vi "ULx Create Channel (AI-Current-Basic).vi"(0 "task in":refnum<k24>, 1 "maximum value":dbl=2.5 format="%_4g", 2 "minimum value":dbl=0.5 format="%_4f", 5 "physical channels":refnum<k21>, 11 "error in":errorcluster) -> (4 "task out":refnum<k24>, 15 "error out":errorcluster)   [LabVIEW 2020]
doc: "Creates channel(s) to measure current."
uses:
  C:/Users/William/Documents/LV 2020 builds/LeaktestDAQ/Source-v33/ULx_LV.dll
  ULx_LV.dll
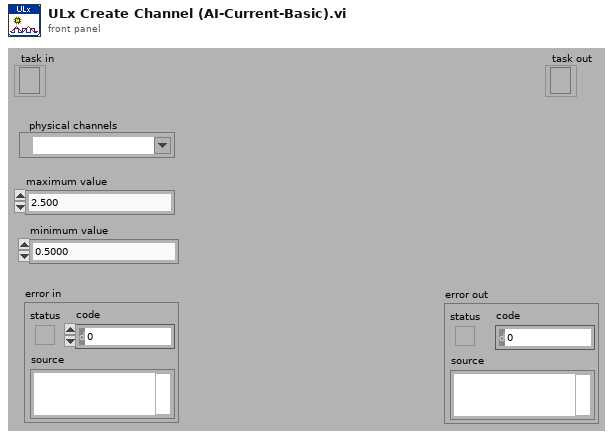
[diagram p1: front panel]
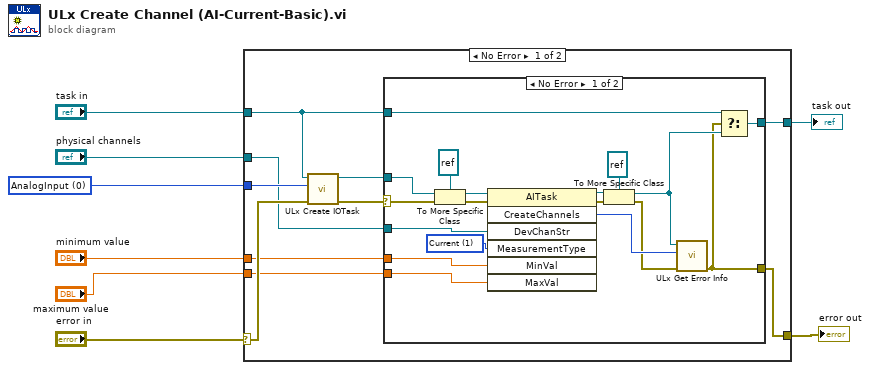
[diagram p0: block diagram]
diagram:
  w2 = 0 items=["AnalogInput", "AnalogOutput", "DigitalInput", "DigitalOutput", "CounterInput", "CounterOutput", "CompositeInput", "CompositeOutput", "TemperatureInput"] ("taskType")
  n1 = case shown="No Error" "error in" {
    selector: "error in" -> [w18 w40]
    tunnel: "task in" -> [w9 w39]
    tunnel: "physical channels" -> [w10 _]
    tunnel: w2 -> [w11 _]
    tunnel: [w16 w39] -> w6
    tunnel: [w15 w40] -> w5
    tunnel: "minimum value" -> [w13 _]
    tunnel: "maximum value" -> [w12 _]
    frame No Error {
      n2 = call "ULx Create IOTask.vi"("error in"=w18, "taskType"=w11, "i/o task in"=w9) -> ("error out"=w17:errorcluster, "i/o task out"=w14:refnum<k24>)  [unwired: 7 in]
      n3 = case shown="No Error" w17 {
        selector: w17 -> [w34 w38]
        tunnel: [w20 w38] -> w15
        tunnel: [w19 w37] -> w16
        tunnel: w14 -> [w32 _]
        tunnel: w10 -> [w31 _]
        tunnel: w13 -> [w29 _]
        tunnel: w12 -> [w28 _]
        tunnel: w9 -> [w22 w37]
        frame No Error {
          w27 = 1 items=["Voltage", "Current"] ("MeasurementType")
          n4 = To More Specific Class(target class=refnum<k24> refnum, reference=w32, error in=w34) -> (specific class reference=w35:refnum<k24>, error out=w33:errorcluster)
          n5 = invoke class="AITask" method="CreateChannels"(reference=w35, error in=w33, "DevChanStr"=w31, "MeasurementType"=w27, "MinVal"=w29, "MaxVal"=w28) -> (reference out=w25:refnum<k24>, error out=w24:errorcluster, "CreateChannels"=w30:i32)  [unwired: 1 in, 4 out]
          n6 = To More Specific Class(target class=refnum<k24> refnum, reference=w25, error in=w24) -> (specific class reference=w21:refnum<k24>, error out=w23:errorcluster)
          n7 = call "ULx Get Error Info.vi"("error in"=w23, "ErrorCode"=w30, "task in"=w21) -> ("error out"=w20:errorcluster)  [unwired: 8 in]
          n8 = Select(t=w22, s=w20, f=w21) -> (s? t:f=w19:refnum<k24>)
        }
        frame Error {
        }
      }
    }
    frame Error {
    }
  }
  "error out" <- w5
  "task out" <- w6
